vi "JKI_Python_Server Example 2 PyObjects 1 Event Structure.vi"() -> ()   [LabVIEW 2013]
uses:
  Server/Register for Events (Multiple PyObjects by Enum).vi
  Server/Server.lvclass
  Call/Call.lvclass
panel:
  in  "Exit":bool
  out "Client Connected":bool
  out "error out":errorcluster
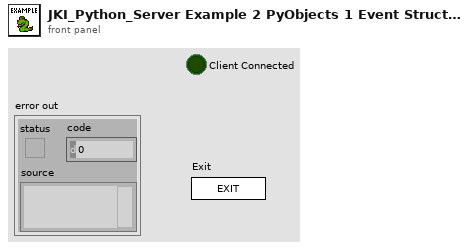
[diagram p1: front panel]
types:
  T1 = enum16{"<unknown python call>", "Object1.HelloWorld", "Object2.Echo", "Object3.Add", "Jim.Test", "Jim.Test2", "Jim.Test3"}
  T2 = typedef "JKI_Python_Bridge_for_LV.lvlib/Server.lvclass/Python Method Call - Event Registration.ctl" = refnum<event-registration>
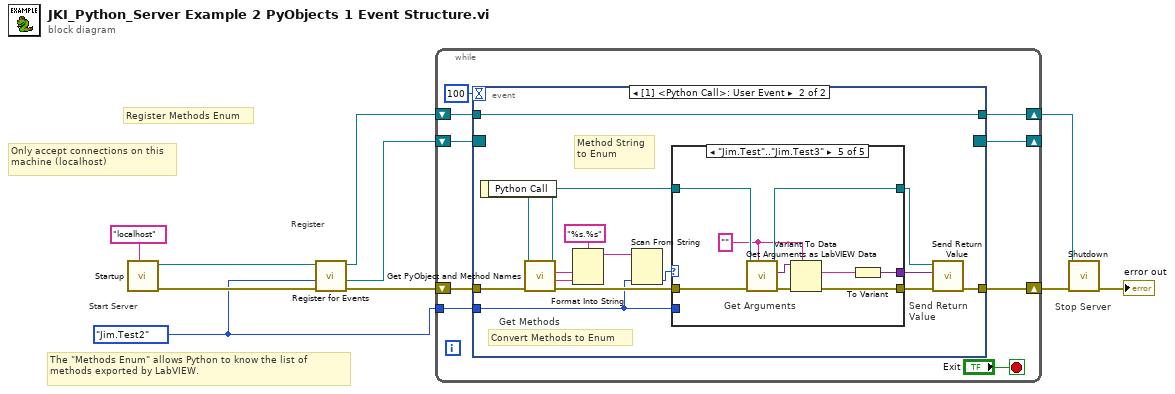
[diagram p0: block diagram]
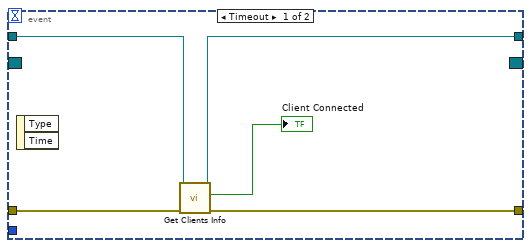
[diagram p2: hidden frame]
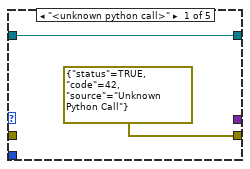
[diagram p3: hidden frame]
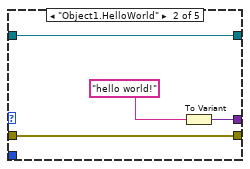
[diagram p4: hidden frame]
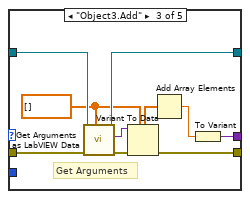
[diagram p5: hidden frame]
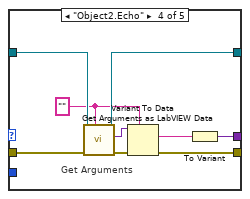
[diagram p6: hidden frame]
diagram:
  w1 = T1."Jim.Test2"
  # "Register"
  # "Stop Server"
  # "Start Server"
  # "The \"Methods Enum\" allows Python to know the list of methods exported by LabVIEW."
  # "Register Methods Enum"
  # "Only accept connections on this machine (localhost)"
  n1 = call "Startup.vi"("IP Address (localhost)"="localhost" ("name")) -> ("error out"=w3:errorcluster, "JKI_Python_Server out"=w8:refnum<class "Server.lvclass">)  [unwired: 9 in]
  n2 = call-poly "Register for Events.vi"("error in (no error)"=w3, "Variant"=w1, "JKI_Python_Server in"=w8) -> ("error out"=w5:errorcluster, "Python"=w2:T2, "JKI_Python_Server out"=w7:refnum<class "Server.lvclass">)  [unwired: 6 in]
  n3 = while {
    shift-right: [w16] -> w4
    shift-left: w5 -> [w18]
    shift-right: [w14] -> w9
    shift-left: w7 -> [w15]
    shift-right: [w13] -> _
    shift-left: w2 -> [w19]
    tunnel: w1 -> [w11]
    stop <- "Exit" stop-if-true
    n4 = event shown="[1] <Python Call>: User Event" {
      selector: w19 -> [_ _]
      dyn-events: [_ _] -> w13
      timeout: 100 -> [_ _]
      tunnel: [w22 w31] -> w16
      tunnel: w18 -> [w23 w36]
      tunnel: w15 -> [w24 w38]
      tunnel: [w20 w38] -> w14
      tunnel: w11 -> [_ w33]
      event Timeout {
        n5 = event-data() -> ()  [unwired: 1 in, 2 out]
        n6 = call "Get Clients Info.vi"("error in (no error)"=w23, "JKI_Python_Server in"=w24) -> ("error out"=w22:errorcluster, "Client Connected"=→"Client Connected":bool, "JKI_Python_Server out"=w20:refnum<class "Server.lvclass">)  [unwired: 5 in, 2 out]
      }
      event User Event {
        # "Convert Methods to Enum"
        # "Send Return\nValue"
        # "Get Methods"
        # "Method String to Enum"
        n7 = event-data() -> ("Python Call"=w37:refnum<class "Call.lvclass">)  [unwired: 1 in]
        n8 = call "Get PyObject and Method Names.vi"("error in (no error)"=w36, "Call in"=w37) -> ("error out"=w35:errorcluster, "Method Name"=w27:string, "PyObject Name"=w28:string, "Call out"=w34:refnum<class "Call.lvclass">)  [unwired: 6 in]
        n9 = Format Into String(format string="%s.%s", w28, w27) -> (resulting string=w25:string)  [unwired: 2 in, 1 out]
        n10 = Scan From String(input string=w25, default 1=w33) -> (output 1=w39:T1)  [unwired: 3 in, 3 out]
        n11 = case shown="\"Jim.Test\"..\"Jim.Test3\"" w39 {
          tunnel: [_ w42 w46 w56 w65] -> w29
          tunnel: w35 -> [_ w44 w49 w60 w69]
          tunnel: [errorcluster {"status"=TRUE, "code"=42, "source"="Unknown Python Call"} ("error out") w44 w54 w64 w73] -> w32
          tunnel: [w41 w43 w51 w62 w71] -> w30
          tunnel: w34 -> [w41 w43 w52 w63 w72]
          tunnel: w33 -> [_ _ _ _ _]
          frame "<unknown python call>" {
          }
          frame "Object1.HelloWorld" {
            n12 = To Variant(anything="hello world!" ("Arguments")) -> (Variant=w42:variant)
          }
          frame "Object3.Add" {
            w47 = dbl[] []
            # "Get Arguments"
            n13 = call "Get Arguments as LabVIEW Data.vi"("type"=w47, "error in (no error)"=w49, "Call in"=w52) -> ("error out"=w48:errorcluster, "LabVIEW Data"=w50:variant, "Call out"=w51:refnum<class "Call.lvclass">)  [unwired: 6 in]
            n14 = Variant To Data(error in=w48, type=w47, Variant=w50) -> (data=w55:dbl[], error out=w54:errorcluster)
            n15 = Add Array Elements(numeric array=w55) -> (sum=w53:dbl)
            n16 = To Variant(anything=w53) -> (Variant=w46:variant)
          }
          frame "Object2.Echo" {
            w58 = ""
            # "Get Arguments"
            n17 = call "Get Arguments as LabVIEW Data.vi"("type"=w58, "error in (no error)"=w60, "Call in"=w63) -> ("error out"=w59:errorcluster, "LabVIEW Data"=w61:variant, "Call out"=w62:refnum<class "Call.lvclass">)  [unwired: 6 in]
            n18 = Variant To Data(error in=w59, type=w58, Variant=w61) -> (data=w57:string, error out=w64:errorcluster)
            n19 = To Variant(anything=w57) -> (Variant=w56:variant)
          }
          frame "Jim.Test".."Jim.Test3" {
            w67 = ""
            # "Get Arguments"
            n20 = call "Get Arguments as LabVIEW Data.vi"("type"=w67, "error in (no error)"=w69, "Call in"=w72) -> ("error out"=w68:errorcluster, "LabVIEW Data"=w70:variant, "Call out"=w71:refnum<class "Call.lvclass">)  [unwired: 6 in]
            n21 = Variant To Data(error in=w68, type=w67, Variant=w70) -> (data=w66:string, error out=w73:errorcluster)
            n22 = To Variant(anything=w66) -> (Variant=w65:variant)
          }
        }
        n23 = call "Send Return Value.vi"("error in (no error)"=w32, "Return Value"=w29, "Response in"=w30) -> ("error out"=w31:errorcluster)  [unwired: 8 in]
      }
    }
  }
  n24 = call "Shutdown.vi"("error in (no error)"=w4, "JKI_Python_Server in"=w9) -> ("error out"=→"error out":errorcluster)  [unwired: 9 in]
